vi "dfd_Find Reciprocal.vi"(10 "zeros out":cdb[](array[numeric]), 11 "zeros in":cdb[](array[numeric])) -> (3 "reciprocal":cdb[](array[numeric]))   [LabVIEW 2017, in "NI_DigFilter_Design.lvlib"]
uses:
  <vilib>/addons/Digital Filter Design/NI_DigFilter_Design.lvlib
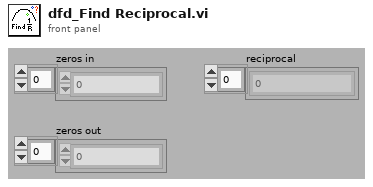
[diagram p1: front panel]
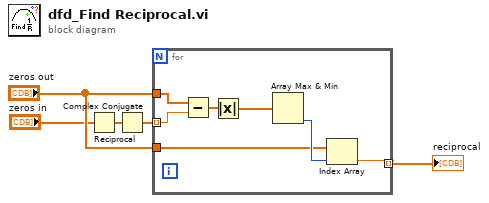
[diagram p0: block diagram]
diagram:
  n1 = Reciprocal(x="zeros in") -> (1/x=w5:cdb[])
  n2 = Complex Conjugate(1:w5) -> (0:w1:cdb[])
  n3 = for {
    tunnel: "zeros out" -> [w7]
    tunnel: w1 -> [w6] mode=indexing
    tunnel: "zeros out" -> [w10]
    tunnel: [w8] -> w2 mode=indexing
    n4 = Subtract(x=w7, y=w6) -> (x-y=w12:cdb[])
    n5 = Absolute Value(x=w12) -> (abs(x)=w9:dbl[])
    n6 = Array Max & Min(array=w9) -> (min index (indices)=w11:i32)  [unwired: 3 out]
    n7 = Index Array(array=w10, index=w11) -> (element=w8:cdb)
  }
  "reciprocal" <- w2
